vi "main 2.18.22 timestamp updated.vi"() -> ()   [LabVIEW 2021]
uses:
  <vilib>/express/express arith-compare/Formula/XNode/ExpressFormulaBlockNode.xnode
  <vilib>/ptbypt/NI_PtbyPt.lvlib
panel:
  out "Waveform Chart 4":waveform(dbl)[](graph)
  in  "Waveform":waveform(dbl)={"t0"=timestamp(0 s since 1904-01-01), "dt"=0.0, "Y"=[]}
  out "Thermistor Filtered":T1(graph)
  out "Thermistor Unfiltered":T1(graph)
  in  "Thermistor":T2
  out "Waveform Chart 3":T3(graph)
  in  "error in (no error)":errorcluster
  out "error out":errorcluster
  out "Waveform Chart 2":waveform(dbl)(graph)
  out "a0 Scalar":dbl
  out "Waveform Chart":dynamicdata(graph)
  in  "stop":bool
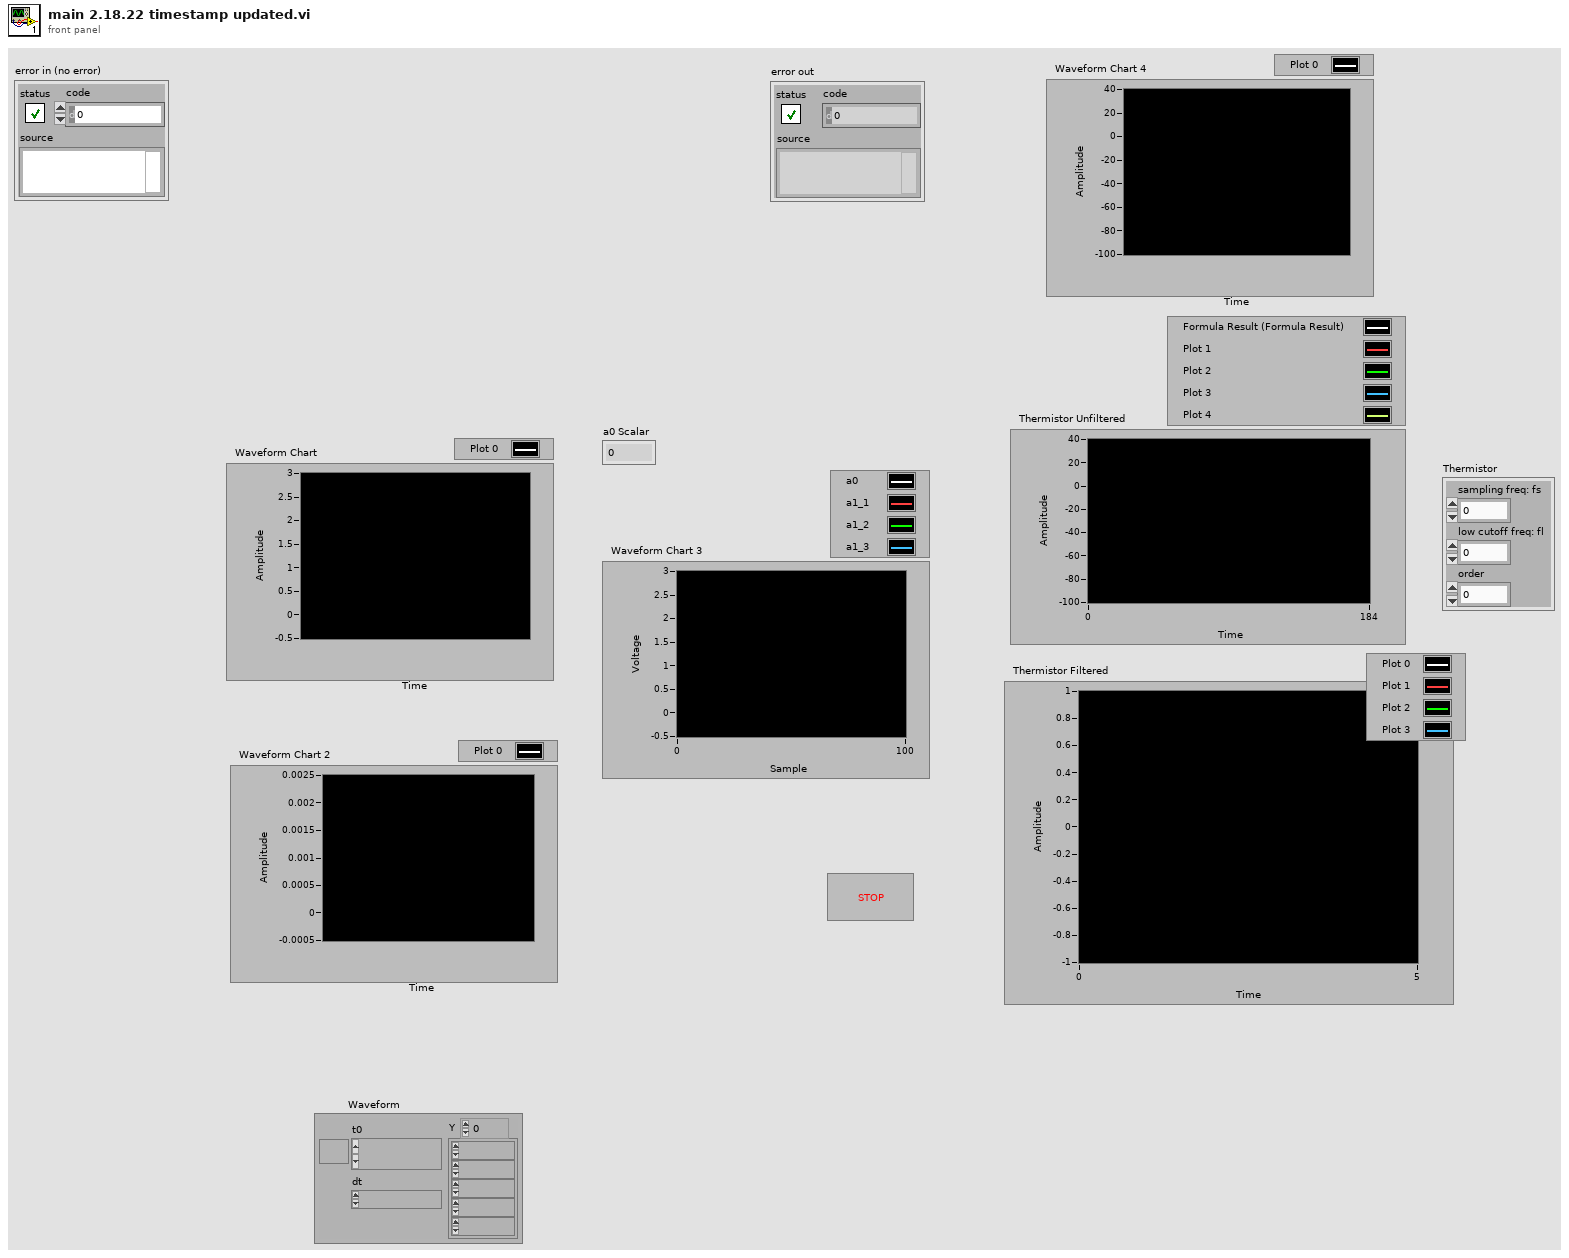
[diagram p1: front panel]
types:
  T1 = cluster{"[0]":dbl, "[1]":dbl, "[2]":dbl, "[3]":dbl, "[4]":dbl, "[5]":dbl, "[6]":dbl, "[7]":dbl, "[8]":dbl}
  T2 = cluster{"sampling freq: fs":dbl, "low cutoff freq: fl":dbl, "order":i32}
  T3 = cluster{"Data_Array[0]":dbl, "Data_Array[1]":dbl, "Data_Array[2]":dbl, "Data_Array[3]":dbl, "Data_Array[4]":dbl, "Data_Array[5]":dbl, "Data_Array[6]":dbl, "Data_Array[7]":dbl, "Data_Array[8]":dbl}
  T4 = cluster{"Data_Array":dbl[], "Multiplex_Tbl":u32[]}
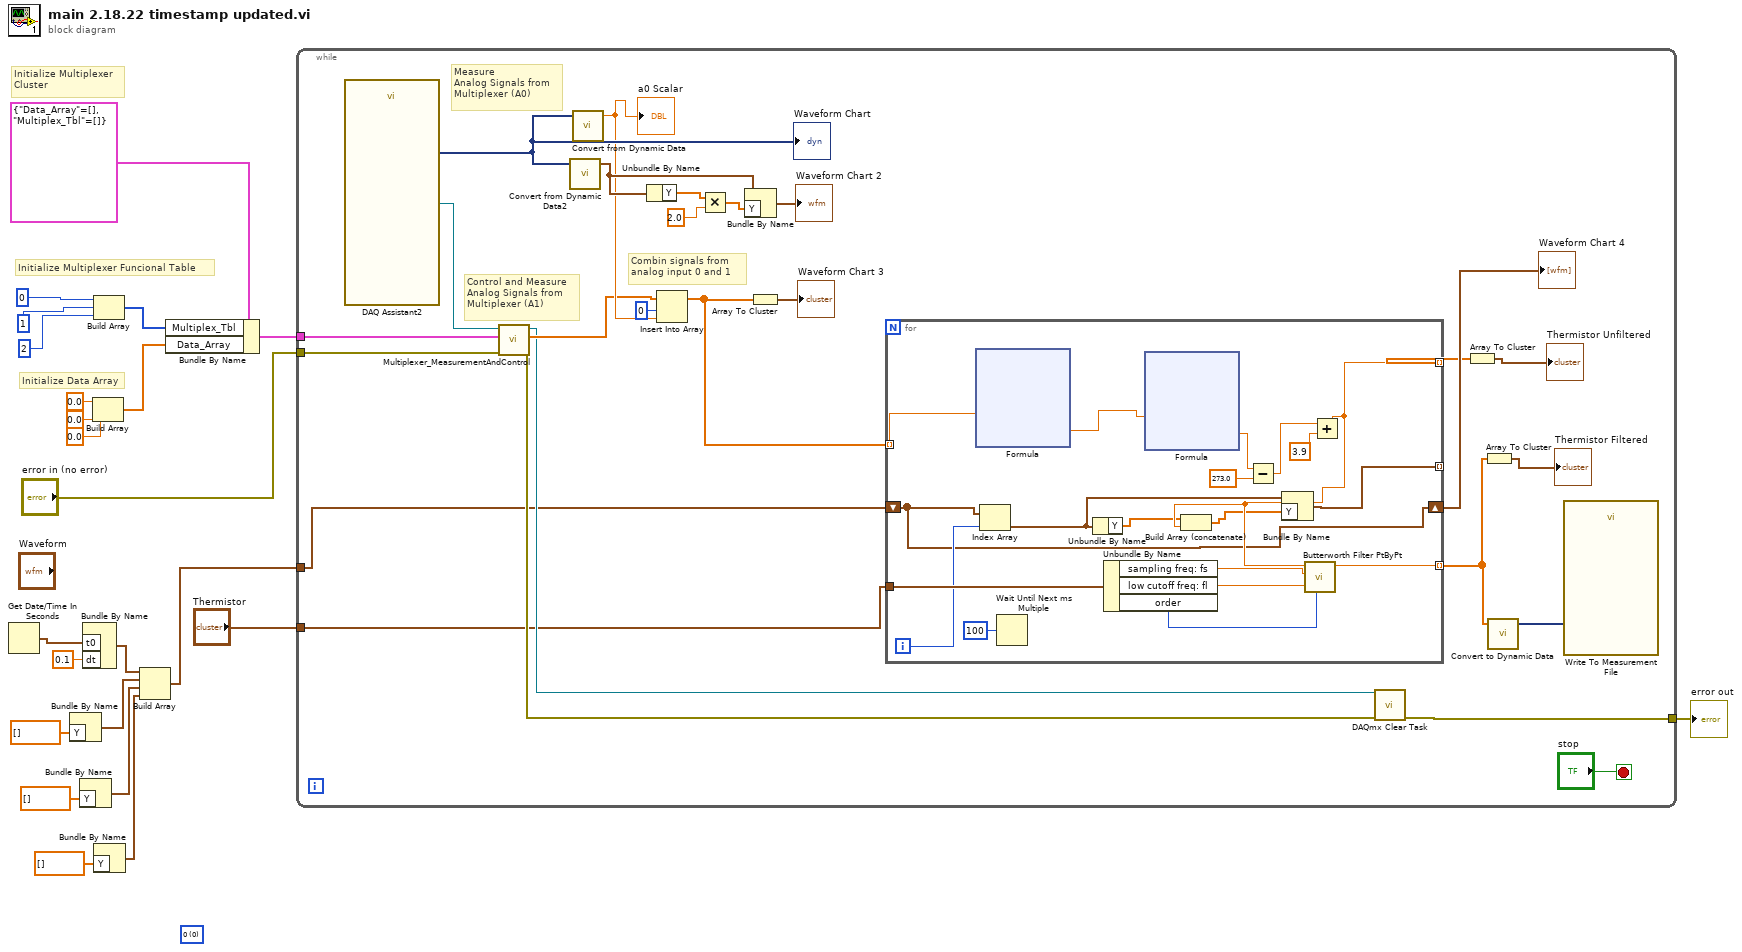
[diagram p0: block diagram]
diagram:
  (unwired) u8 0 items=["0", "1", "Z", "L", "H", "X", "T", "V"] ("digital values ring")
  # "Initialize Multiplexer \nCluster"
  # "Initialize Data Array"
  # "Initialize Multiplexer Funcional Table"
  n1 = Get Date/Time In Seconds() -> (seconds since 1Jan1904=w10:timestamp)
  n2 = Bundle By Name("Y"=dbl[] []) -> (w5:waveform(dbl))  [unwired: 1 in]
  n3 = Bundle By Name("Y"=dbl[] []) -> (w2:waveform(dbl))  [unwired: 1 in]
  n4 = Bundle By Name("t0"=w10, "dt"=0.1) -> (w8:waveform(dbl))  [unwired: 1 in]
  n5 = Build Array(0.0 ("element"), 0.0 ("element"), 0.0 ("element")) -> (w19:dbl[])
  n6 = Build Array(u32 0 ("Waveform"), 1 ("Waveform"), u32 2 ("Waveform")) -> (w13:u32[])
  n7 = Bundle By Name("Y"=dbl[] []) -> (w1:waveform(dbl))  [unwired: 1 in]
  n8 = Build Array(w8, w5, w2, w1) -> (w7:waveform(dbl)[])
  n9 = Bundle By Name(cluster=T4 {"Data_Array"=[], "Multiplex_Tbl"=[]}, "Multiplex_Tbl"=w13, "Data_Array"=w19) -> (w18:T4)
  n10 = while {
    tunnel: w18 -> [w42]
    tunnel: "error in (no error)" -> [w41]
    tunnel: [w33] -> w12
    tunnel: "Thermistor" -> [w32]
    tunnel: w7 -> [w27]
    stop <- "stop" stop-if-true
    # "Combin signals from \nanalog input 0 and 1"
    # "Measure\nAnalog Signals from\nMultiplexer (A0)"
    # "Control and Measure\nAnalog Signals from\nMultiplexer (A1)"
    n11 = call "DAQ Assistant2"() -> ("task out"=w40:refnum<k21>, "data"=w43:dynamicdata)  [unwired: 16 in, 2 out]
    "Waveform Chart" <- w43
    n12 = call "Multiplexer_MeasurementAndControl.vi"("error in (no error)"=w41, "Multiplexer_Cluser"=w42, "Task in"=w40) -> ("error out"=w34:errorcluster, "Data_Array"=w37:dbl[], "Task out"=w35:refnum<k21>)  [unwired: 6 in]
    n13 = call "Convert from Dynamic Data2"("Dynamic Data Type"=w43) -> ("Waveform"=w46:waveform(dbl))  [unwired: 3 in]
    n14 = call "Convert from Dynamic Data"("Dynamic Data Type"=w43) -> ("Scalar"=w39:dbl)  [unwired: 3 in]
    "a0 Scalar" <- w39
    n15 = Unbundle By Name(w46) -> ("Y"=w48:dbl[])
    n16 = Insert Into Array(array=w37, index=0, new element=w39) -> (w31:dbl[])
    n17 = Multiply(x=w48, y=2.0) -> (x*y=w45:dbl[])
    n18 = Bundle By Name(cluster=w46, "Y"=w45) -> (→"Waveform Chart 2":waveform(dbl))
    n19 = Array To Cluster(array=w31) -> (cluster=→"Waveform Chart 3":T3)
    n20 = for {
      tunnel: w31 -> [w61] mode=indexing
      tunnel: w32 -> [w60]
      tunnel: [w56] -> w24 mode=indexing
      tunnel: [w59] -> w29 mode=indexing
      shift-right: [w50] -> w26
      shift-left: w27 -> [w50]
      tunnel: [w51] -> _ mode=indexing
      i -> [w53]
      n21 = xnode "Formula"("v"=w61) -> ("Result"=w67:dbl)  [unwired: 1 in, 1 out]
      n22 = Index Array(array=w50, index=w53) -> (element=w52:waveform(dbl))
      n23 = Wait Until Next ms Multiple(millisecond multiple=u32 100) -> ()  [unwired: 1 out]
      n24 = Unbundle By Name(w52) -> ("Y"=w55:dbl[])
      n25 = Unbundle By Name(w60) -> ("sampling freq: fs"=w66:dbl, "low cutoff freq: fl"=w65:dbl, "order"=w64:i32)
      n26 = xnode "Formula"("R"=w67) -> ("Result"=w62:dbl)  [unwired: 1 in, 1 out]
      n27 = Subtract(x=w62, y=273.0) -> (x-y=w57:dbl)
      n28 = Add(x=w57, y=3.9) -> (x+y=w56:dbl)
      n29 = Build Array (concatenate)(w55, w56) -> (w54:dbl[])
      n30 = Bundle By Name(cluster=w52, "Y"=w54) -> (w51:waveform(dbl))
      n31 = call <vilib>:"Butterworth Filter PtByPt.vi"("order"=w64, "low cutoff freq: fl"=w65, "sampling freq: fs"=w66, "x"=w56) -> ("Filtered x"=w59:dbl)  [unwired: 5 in, 1 out]
    }
    "Waveform Chart 4" <- w26
    n32 = call <vilib>:"DAQmx Clear Task.vi"("task in"=w35, "error in"=w34) -> ("error out"=w33:errorcluster)  [unwired: 13 in]
    n33 = Array To Cluster(array=w24) -> (cluster=→"Thermistor Unfiltered":T1)
    n34 = Array To Cluster(array=w29) -> (cluster=→"Thermistor Filtered":T1)
    n35 = call "Convert to Dynamic Data"("Array"=w29) -> ("Dynamic Data Type"=w30:dynamicdata)  [unwired: 3 in]
    n36 = call "Write To Measurement File"("Signals"=w30) -> ()  [unwired: 16 in, 3 out]
  }
  "error out" <- w12
